vi "Teardown.vi"(8 "error in (no error)":errorcluster, 11 "Bus Monitor in":refnum<class "Bus Monitor.lvclass">) -> (0 "error out":errorcluster)   [LabVIEW 2020, in "Unit Tests.lvlib" / "Bus Monitor.lvclass"]
uses:
  Bus Monitor.lvclass
  Utilities/Simulated FPGA/FPGA Sim.lvclass
  Bus Monitor.lvclass/Bus Monitor.ctl
  1553 Session/1553 Session.lvclass
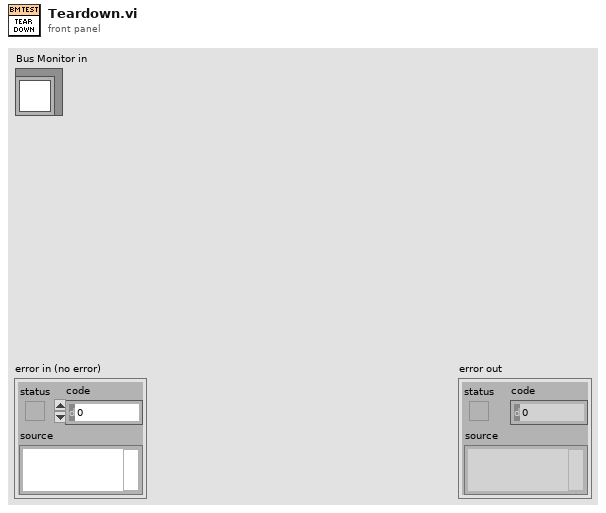
[diagram p1: front panel]
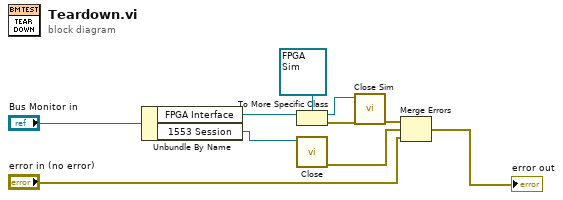
[diagram p0: block diagram]
diagram:
  n1 = Unbundle By Name("Bus Monitor in") -> ("FPGA Interface"=w4:refnum<class "FPGA Interface.lvclass">, "1553 Session"=w3:refnum<class "1553 Session.lvclass">)
  n2 = To More Specific Class(target class=refnum<class "FPGA Sim.lvclass"> refnum ("FPGA Sim.lvclass"), reference=w4) -> (specific class reference=w6:refnum<class "FPGA Sim.lvclass">, error out=w5:errorcluster)  [unwired: 1 in]
  n3 = call-dynamic "Close.vi"("1553 Board in"=w3) -> ("error out"=w1:errorcluster)  [unwired: 10 in]
  n4 = call "Close Sim.vi"("error in (no error)"=w5, "FPGA Sim in"=w6) -> ("error out"=w2:errorcluster)  [unwired: 9 in]
  n5 = Merge Errors(w2, w1, "error in (no error)") -> (→"error out":errorcluster)
